vi "Get Position Deadband.vi"(4 "error in (no error)":errorcluster, 6 "Axis (1)":i32=1 min=0 max=3, 7 "VISA resource name":refnum<visa-resource-name>) -> (0 "error out":errorcluster, 2 "Deadband (encoder counts)":i32, 3 "VISA resource name out":refnum<visa-resource-name>)   [LabVIEW 2019, in "Newport ESP301.lvlib"]
doc: "Reads the position deadband value for an axis"
uses:
  Newport ESP301.lvlib
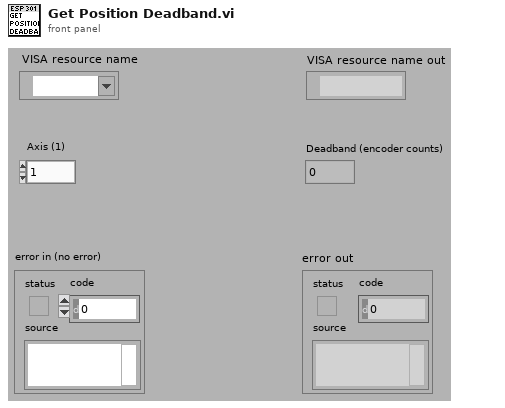
[diagram p1: front panel]
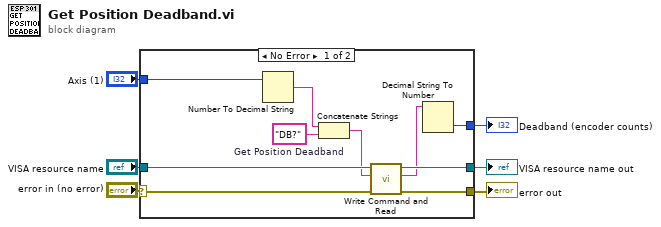
[diagram p0: block diagram]
diagram:
  n1 = case shown="No Error" "error in (no error)" {
    selector: "error in (no error)" -> [w13 w18]
    tunnel: [w15 w18] -> w6
    tunnel: "VISA resource name" -> [w16 w17]
    tunnel: [w14 w17] -> w5
    tunnel: [w12 _] -> w1
    tunnel: "Axis (1)" -> [w9 _]
    frame No Error {
      w11 = "DB?"  # Get Position Deadband
      n2 = Number To Decimal String(number=w9) -> (decimal integer string=w10:string)  [unwired: 1 out]
      n3 = Concatenate Strings(w10, w11) -> (w8:string)
      n4 = call "Write Command and Read.vi"("error in (no error)"=w13, "Command"=w8, "VISA resource name"=w16) -> ("error out"=w15:errorcluster, "Returned string"=w7:string, "VISA resource name out"=w14:refnum<visa-resource-name>)  [unwired: 2 in, 2 out]
      n5 = Decimal String To Number(string=w7) -> (number=w12:i32)  [unwired: 3 out]
    }
    frame Error {
    }
  }
  "error out" <- w6
  "VISA resource name out" <- w5
  "Deadband (encoder counts)" <- w1
